vi "Read Power W Averaging.vi"(6 "Index In":u32, 7 "Buffer In":dbl[](array[numeric]), 8 "error in (no error)":errorcluster, 10 "VISA Resource Name":refnum<visa-resource-name>, 11 "Cluster In":T2={"Wavelength"=0.0, "AVG"=0, "Range"=0, "Backlight"=0, "Beeper"=0, "Zero"=0, "Local Lockout"=0, "ATTN"=0, "Run/Stop"=0, "Units"=0, "Averaging Points"=0, "Averaging"=FALSE, "Most Recent Power"=5.5, "Filter"=1} {"AVG" items=["Slow"=1, "Medium"=2, "Fast"=3]; "Range" items=["Auto", "Lowest", "2", "3", "4", "5", "6", "7", "Highest"]; "Backlight" items=["Off", "Low", "High"]; "Beeper" items=["Off", "On"]; "Zero" items=["Off", "On"]; "Local Lockout" items=["Off", "On"]; "ATTN" items=["Off", "On"]; "Run/Stop" items=["Stop", "Run"]; "Units" items=["W"=1, "dB"=2, "dBm"=3, "REL"=4]; "Filter" items=["Orange"=1, "Green"=2, "Yellow"=3]}) -> (0 "error out":errorcluster, 1 "Current Power w/ Units":string, 2 "Current Power":dbl[unit], 3 "Cluster Out":T2={"Wavelength"=0.0, "AVG"=0, "Range"=0, "Backlight"=0, "Beeper"=0, "Zero"=0, "Local Lockout"=0, "ATTN"=0, "Run/Stop"=0, "Units"=0, "Averaging Points"=0, "Averaging"=FALSE, "Most Recent Power"=5.5, "Filter"=1} {"AVG" items=["Slow"=1, "Medium"=2, "Fast"=3]; "Range" items=["Auto", "Lowest", "2", "3", "4", "5", "6", "7", "Highest"]; "Backlight" items=["Off", "Low", "High"]; "Beeper" items=["Off", "On"]; "Zero" items=["Off", "On"]; "Local Lockout" items=["Off", "On"]; "ATTN" items=["Off", "On"]; "Run/Stop" items=["Stop", "Run"]; "Units" items=["W"=1, "dB"=2, "dBm"=3, "REL"=4]; "Filter" items=["Orange"=1, "Green"=2, "Yellow"=3]}, 4 "Index Out":u32, 5 "Buffer Out":dbl[](array[numeric]))   [LabVIEW 2013]
doc: "Advanced Read for Power Meter.\n\nPerforms time-based Averaging based of member data. Checks for erroneous data points due to auto-ranging. Also has formatted power output."
uses:
  Public/Filters.ctl
  Newport 1830-C.lvlib
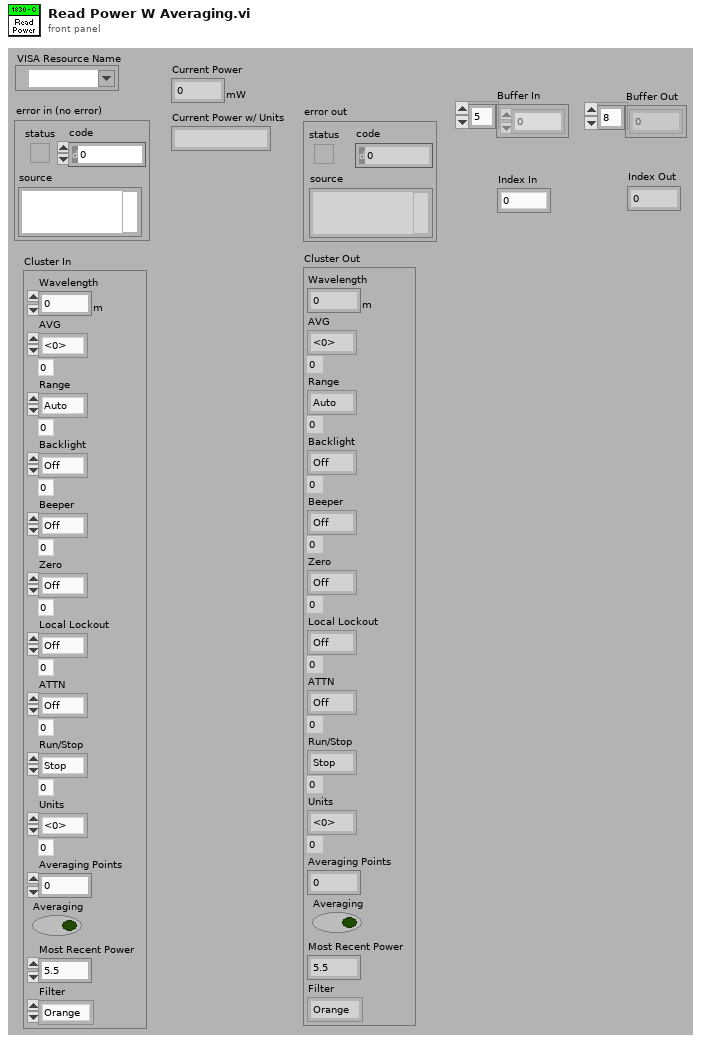
[diagram p1: front panel]
types:
  T1 = typedef "Newport 1830-C.lvlib/Filters.ctl" = u16
  T2 = cluster{"Wavelength":dbl[unit], "AVG":u16, "Range":u16, "Backlight":u16, "Beeper":u16, "Zero":u16, "Local Lockout":u16, "ATTN":u16, "Run/Stop":u16, "Units":u16, "Averaging Points":u32, "Averaging":bool, "Most Recent Power":dbl, "Filter":T1}
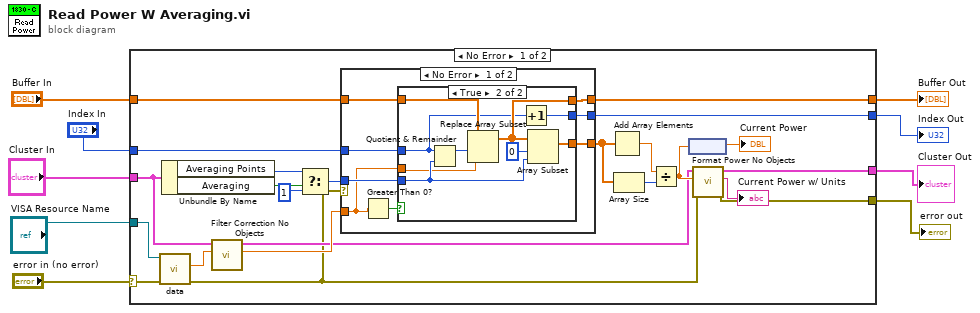
[diagram p0: block diagram]
diagram:
  n1 = case shown="No Error" "error in (no error)" {
    selector: "error in (no error)" -> [w17 w57]
    tunnel: [w24 w57] -> w9
    tunnel: [w25 w56] -> w7
    tunnel: "VISA Resource Name" -> [w23 _]
    tunnel: "Cluster In" -> [w22 w56]
    tunnel: [w16 w55] -> w5
    tunnel: "Buffer In" -> [w15 w55]
    tunnel: "Index In" -> [w14 w54]
    tunnel: [w13 w54] -> w2
    frame No Error {
      n2 = call "data.vi"("error in (no error)"=w17, "VISA resource name"=w23) -> ("error out"=w10:errorcluster, "Power"=w21:dbl)  [unwired: 7 in, 1 out]
      n3 = Unbundle By Name(w22) -> ("Averaging Points"=w11:u32, "Averaging"=w28:bool)
      n4 = call "Filter Correction No Objects.vi"("Read Power"=w21, "Cluster In"=w22) -> ("Corrected Power"=w20:dbl, "Cluster Out"=w12:T2)  [unwired: 8 in]
      n5 = Select(t=w11, s=w28, f=u32 1 ("t")) -> (s? t:f=w19:u32)
      n6 = case shown="No Error" w10 {
        tunnel: w20 -> [w34 _]
        tunnel: w19 -> [w40 _]
        tunnel: [w39 w52] -> w18
        tunnel: [w38 w52] -> w16
        tunnel: w15 -> [w37 w52]
        tunnel: w14 -> [w36 w53]
        tunnel: [w35 w53] -> w13
        frame No Error {
          n7 = Greater Than 0?(x=w34) -> (x > 0?=w33:bool)
          n8 = case shown="True" w33 {
            tunnel: w40 -> [_ w51]
            tunnel: [w41 w50] -> w39
            tunnel: [w41 w49] -> w38
            tunnel: w37 -> [w41 w48]
            tunnel: w36 -> [w42 w47]
            tunnel: [w42 w46] -> w35
            tunnel: w34 -> [_ w43]
            frame False {
            }
            frame True {
              n9 = Quotient & Remainder(x=w47, y=w51) -> (x-y*floor(x/y)=w45:u32)  [unwired: 1 out]
              n10 = Replace Array Subset(array=w48, new element=w43, index=w45) -> (w49:dbl[])
              n11 = Increment(x=w47) -> (x+1=w46:u32)
              n12 = Array Subset(array=w49, index=0, length=w51) -> (w50:dbl[])
            }
          }
        }
        frame Error {
        }
      }
      n13 = Add Array Elements(numeric array=w18) -> (sum=w30:dbl)
      n14 = Array Size(array=w18) -> (size(s)=w31:i32)
      n15 = Divide(x=w30, y=w31) -> (x/y=w27:dbl)
      n16 = node(w27) -> (→"Current Power":dbl[unit])
      n17 = call "Format Power No Objects.vi"("error in"=w10, "Power"=w27, "Cluster In"=w12) -> ("error out"=w24:errorcluster, "Formatted Power"=→"Current Power w/ Units":string, "Cluster Out"=w25:T2)  [unwired: 6 in]
    }
    frame Error {
    }
  }
  "error out" <- w9
  "Cluster Out" <- w7
  "Buffer Out" <- w5
  "Index Out" <- w2
